vi "Resistance_test_2.vi"() -> ()   [LabVIEW 2017]
uses:
  <vilib>/DAQmx/write.llb/DAQmx Write (Analog DBL 1Chan 1Samp).vi
  <vilib>/DAQmx/create/channels.llb/DAQmx Create Channel (AI-Voltage-Basic).vi
  <vilib>/DAQmx/create/channels.llb/DAQmx Create Channel (AO-Voltage-Basic).vi
  <vilib>/DAQmx/miscellaneous.llb/DAQmx Fill In Error Info.vi
panel:
  out "Voltage graph":cluster{dbl[], dbl[]}(graph)
  out "Resistance graph":cluster{dbl[], dbl[]}(graph)
  out "Voltage":dbl
  out "Average Voltage U, V":dbl
  in  "time delay, ms":u32=100
  out "Average resistance, Ohm":dbl=0.9828221329838531
  in  "DAQ channel In Voltage Output":tag="DAQ6363/ao0"
  out "error out":errorcluster
  in  "Voltage Output, V":dbl=1.0 min=0.0 max=10.0 format="%#.2f"
  in  "Averaging points":i32=100
  in  "Rsh, Ohm":dbl=5091.0 min=0.0
  in  "Error In (no error)":errorcluster
  in  "DAQ channel In Voltage U":tag="DAQ6363/ai5"
  in  "DAQ channel In Voltage Ush":tag="DAQ6363/ai4"
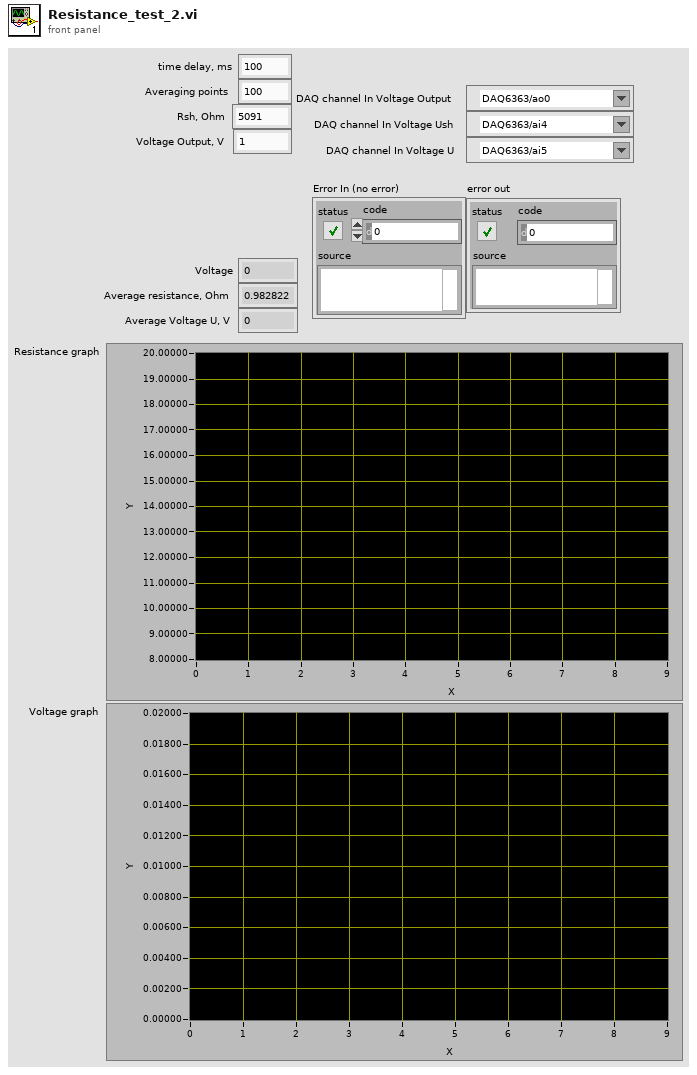
[diagram p1: front panel]
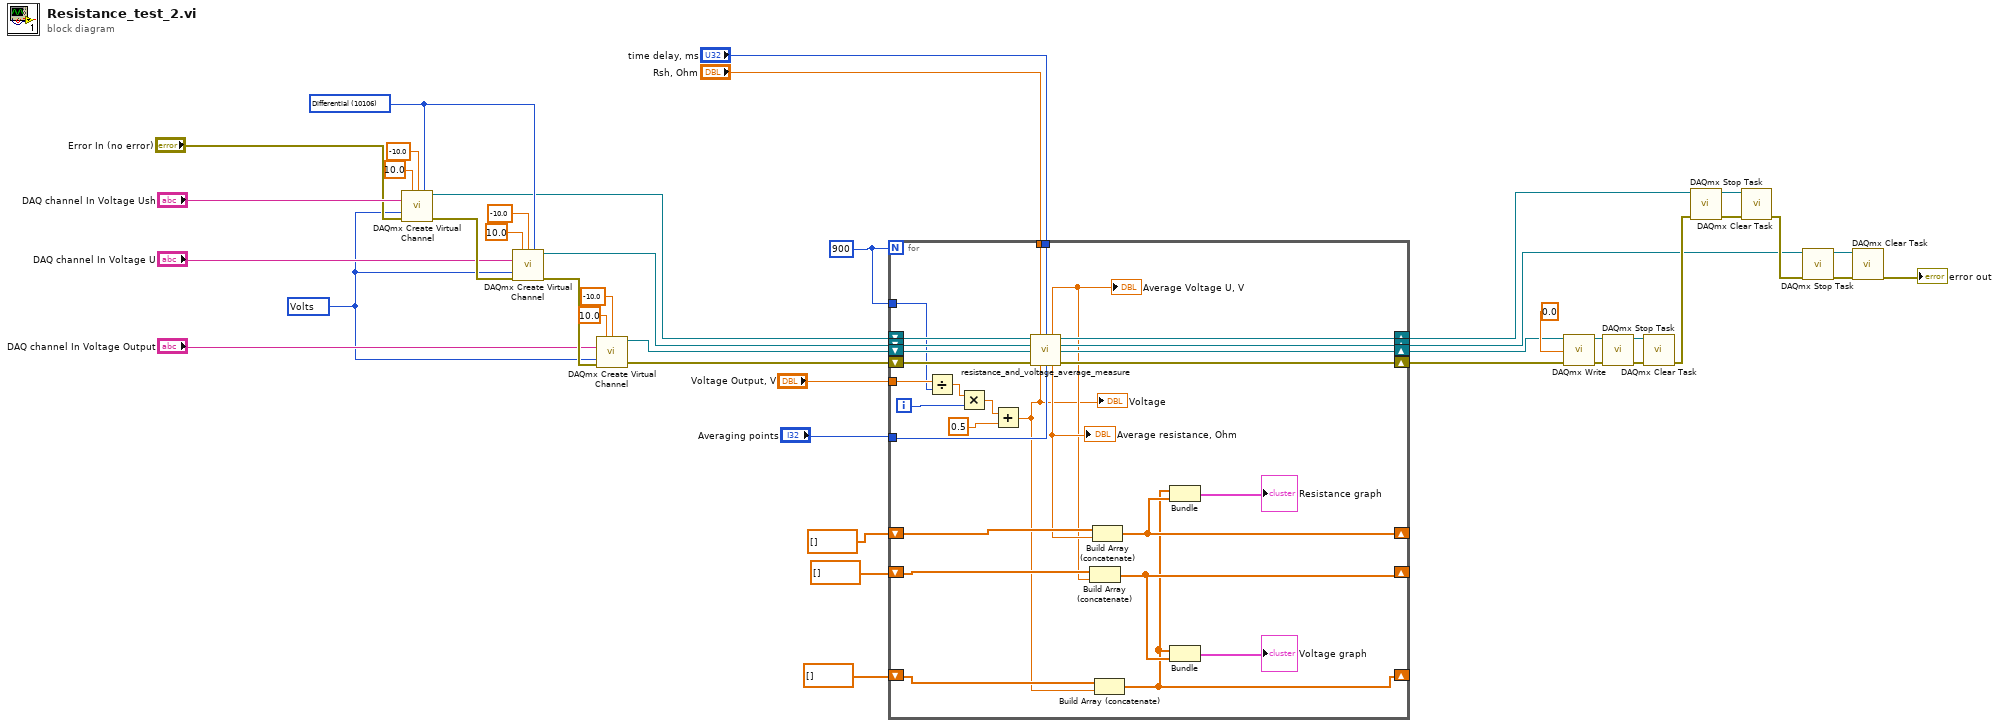
[diagram p0: block diagram]
diagram:
  w4 = 900
  w23 = 10106 items=["Default"=-1, "RSE"=10083, "NRSE"=10078, "Differential"=10106, "Pseudodifferential"=12529] ("input terminal configuration")
  w24 = 10348 items=["Volts"=10348, "From Custom Scale"=10065] ("units")
  n1 = call-poly <vilib>:"DAQmx Create Virtual Channel.vi"("maximum value"=10.0, "minimum value"=-10.0, "input terminal configuration"=w23, "physical channels"="DAQ channel In Voltage Ush", "units"=w24, "error in"="Error In (no error)") -> ("task out"=w16:refnum<k21>, "error out"=w42:errorcluster)  [unwired: 8 in]
  n2 = call-poly <vilib>:"DAQmx Create Virtual Channel.vi"("maximum value"=10.0, "minimum value"=-10.0, "input terminal configuration"=w23, "physical channels"="DAQ channel In Voltage U", "units"=w24, "error in"=w42) -> ("task out"=w15:refnum<k21>, "error out"=w32:errorcluster)  [unwired: 8 in]
  n3 = call-poly <vilib>:"DAQmx Create Virtual Channel.vi"("maximum value"=10.0, "minimum value"=-10.0, "physical channels"="DAQ channel In Voltage Output", "units"=w24, "error in"=w32) -> ("task out"=w14:refnum<k21>, "error out"=w13:errorcluster)  [unwired: 9 in]
  n4 = for {
    N: w4 -> [_]
    tunnel: "Rsh, Ohm" -> [w62]
    tunnel: "time delay, ms" -> [w61]
    tunnel: "Voltage Output, V" -> [w59]
    tunnel: "Averaging points" -> [w60]
    shift-right: [w63] -> w9
    shift-left: w16 -> [w70]
    shift-right: [w64] -> w10
    shift-left: w15 -> [w69]
    shift-right: [w65] -> w11
    shift-left: w14 -> [w68]
    shift-right: [w66] -> w12
    shift-left: w13 -> [w67]
    tunnel: w4 -> [w58]
    shift-right: [w50] -> _
    shift-left: dbl[] [] -> [w55]
    shift-right: [w48] -> _
    shift-left: dbl[] [] -> [w53]
    shift-right: [w46] -> _
    shift-left: dbl[] [] -> [w47]
    i -> [w57]
    n5 = Divide(x=w59, y=w58) -> (x/y=w56:dbl)
    n6 = Multiply(x=w56, y=w57) -> (x*y=w44:dbl)
    n7 = Add(x=w44, y=0.5) -> (x+y=w43:dbl)
    "Voltage" <- w43
    n8 = call "resistance_and_voltage_average_measure.vi"("DAQ task Voltage Ush (in)"=w70, "Rsh, Ohm"=w62, "time delay, ms"=w61, "DAQ task Voltage U (in)"=w69, "DAQ task Voltage Output (in)"=w68, "error in (no error)"=w67, "Voltage Output, V"=w43, "Averaging points"=w60) -> ("Average Voltage, V"=w52:dbl, "DAQ task Voltage Ush (out)"=w63:refnum<k21>, "DAQ task Voltage U (out)"=w64:refnum<k21>, "DAQ task Voltage Output (out)"=w65:refnum<k21>, "Average Resistance, Ohm"=w54:dbl, "error out"=w66:errorcluster)  [unwired: 2 in]
    "Average resistance, Ohm" <- w54
    "Average Voltage U, V" <- w52
    n9 = Build Array (concatenate)(w53, w52) -> (w48:dbl[])
    n10 = Build Array (concatenate)(w55, w54) -> (w50:dbl[])
    n11 = Build Array (concatenate)(w47, w43) -> (w46:dbl[])
    n12 = Bundle(w46, w50) -> (→"Resistance graph":cluster{dbl[], dbl[]})  [unwired: 1 in]
    n13 = Bundle(w46, w48) -> (→"Voltage graph":cluster{dbl[], dbl[]})  [unwired: 1 in]
  }
  n14 = call-poly <vilib>:"DAQmx Write.vi"("task/channels in"=w11, "data"=0.0, "error in"=w12) -> ("task out"=w28:refnum<k21>, "error out"=w26:errorcluster)  [unwired: 10 in, 1 out]
  n15 = call <vilib>:"DAQmx Stop Task.vi"("task/channels in"=w28, "error in"=w26) -> ("task out"=w30:refnum<k21>, "error out"=w29:errorcluster)  [unwired: 12 in]
  n16 = call <vilib>:"DAQmx Clear Task.vi"("task in"=w30, "error in"=w29) -> ("error out"=w25:errorcluster)  [unwired: 13 in]
  n17 = call <vilib>:"DAQmx Stop Task.vi"("task/channels in"=w9, "error in"=w25) -> ("task out"=w40:refnum<k21>, "error out"=w39:errorcluster)  [unwired: 12 in]
  n18 = call <vilib>:"DAQmx Clear Task.vi"("task in"=w40, "error in"=w39) -> ("error out"=w36:errorcluster)  [unwired: 13 in]
  n19 = call <vilib>:"DAQmx Stop Task.vi"("task/channels in"=w10, "error in"=w36) -> ("task out"=w37:refnum<k21>, "error out"=w38:errorcluster)  [unwired: 12 in]
  n20 = call <vilib>:"DAQmx Clear Task.vi"("task in"=w37, "error in"=w38) -> ("error out"=→"error out":errorcluster)  [unwired: 13 in]
